vi "Launch Logger if Configured.vi"(8 "error in (no error)":errorcluster, 11 "Historian Module in":refnum<class "Historian Module.lvclass">) -> (0 "error out":errorcluster, 3 "Historian Module out":refnum<class "Historian Module.lvclass">)   [LabVIEW 2020, in "VolatusHistorian.lvlib" / "Historian Module.lvclass"]
uses:
  Historian Module.lvclass
  C:/dev/lv20CE/relink/lv-volatus/Volatus/Module/Module.lvclass
  Volatus/Module/Module.lvclass/Module.ctl
  VolatusConfig/VolatusConfigElement/VolatusConfigElement.lvclass/VolatusConfigElement.ctl
  Volatus/Module/Config.vi
  VolatusConfig/VolatusConfigElement/Element.vi
  VolatusConfig/Task/Task Config.lvclass
  C:/dev/lv20CE/relink/lv-volatus/VolatusConfig/VolatusConfigElement/VolatusConfigElement.lvclass
  Historian Module.lvclass/Historian Module.ctl
  Volatus/Module/Module.lvclass
  VolatusConfig/VolatusConfigElement/VolatusConfigElement.lvclass
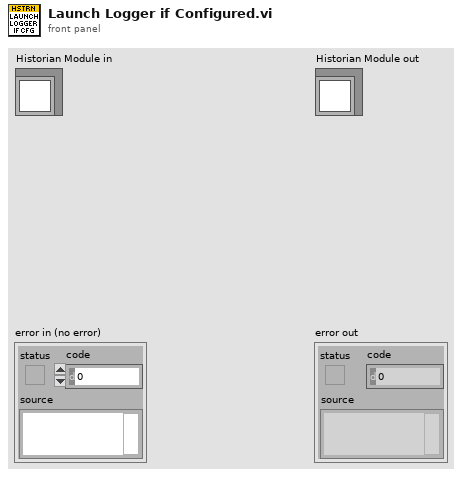
[diagram p1: front panel]
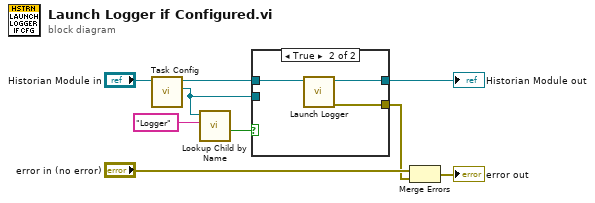
[diagram p0: block diagram]
diagram:
  n1 = call "Task Config.vi"("Module in"="Historian Module in") -> ("Task Config"=w4:refnum<class "Task Config.lvclass">, "Module out"=w6:refnum<class "Historian Module.lvclass">)  [unwired: 8 in, 1 out]
  n2 = call "Lookup Child by Name.vi"("Child Name"="Logger", "VolatusConfigElement in"=w4) -> ("Found"=w5:bool)  [unwired: 6 in, 3 out]
  n3 = case shown="True" w5 {
    tunnel: w6 -> [w10 w13]
    tunnel: w4 -> [_ _]
    tunnel: [w10 w12] -> w3
    tunnel: [_ w11] -> w1
    frame False {
      # "Historian Logger not configured"
    }
    frame True {
      n4 = call "Launch Logger.vi"("Historian Module in"=w13) -> ("error out"=w11:errorcluster, "Historian Module out"=w12:refnum<class "Historian Module.lvclass">)  [unwired: 9 in]
    }
  }
  "Historian Module out" <- w3
  n5 = Merge Errors("error in (no error)", w1) -> (→"error out":errorcluster)
